vi "stop robot move.vi"   [LabVIEW 2018]
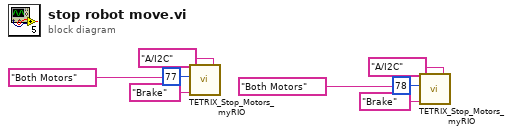
[diagram p0: block diagram]
diagram:
  n1 = call <vilib>:"TETRIX_Stop_Motors_myRIO.vi"("myRIO MXP Port A/B"=tag "A/I2C", "Stop Mode"="Brake", "Select Channel"="Both Motors", "Controller ID#  (I2C Address)"=u8 77) -> ()  [unwired: 3 in, 1 out]
  n2 = call <vilib>:"TETRIX_Stop_Motors_myRIO.vi"("myRIO MXP Port A/B"=tag "A/I2C", "Stop Mode"="Brake", "Select Channel"="Both Motors", "Controller ID#  (I2C Address)"=u8 78) -> ()  [unwired: 3 in, 1 out]
